vi "WILT Panel SS Station Labels.vi"(10 "Label Com Array":string[][](array[string])=[["M1", "100"], ["M3", "3"], ["M5", "5"], ["M7", "7"], ["M9", "9"], ["M11", "11"], ["M13", "13"], ["M15", "15"], ["M17", "17"], ["M19", "19"], ["M2", "2"], ["M4", "4"], ["M6", "6"], ["M8", "8"], ["M10", "10"], ["M12", "12"], ["M14", "14"], ["M16", "16"], ["M18", "18"], ["M20", "20"], ["N6", "21"], ["N7", "22"], ["N8", "23"], ["N9", "24"], ["N10", "25"], ["N11", "26"], ["N12", "27"], ["N13", "28"]]) -> (2 "Array Out":string[][](array[string]))   [LabVIEW 2016]
panel:
  in  "Complete":bool
  in  "Station A":string="DGnn"
  in  "Station C":string="58,50"
  in  "Station D":string="GE HEWH 1"
  in  "Station B":string="HEWH-MAN_OV"
  # "Enter Station Labels"
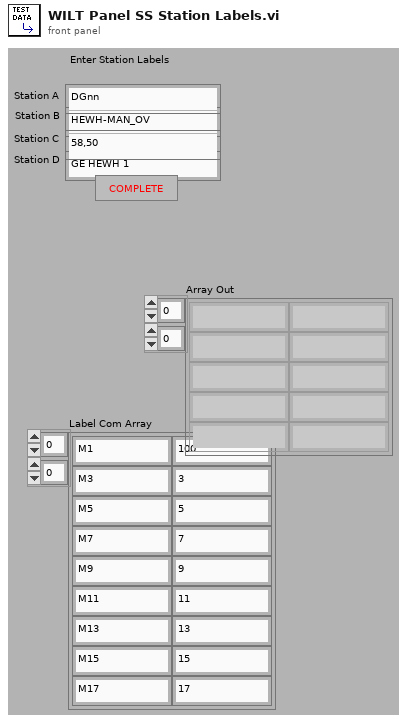
[diagram p1: front panel]
types:
  T1 = cluster{"Label Com Array[0]":string, "Label Com Array[1]":string, "Label Com Array[2]":string, "Label Com Array[3]":string}
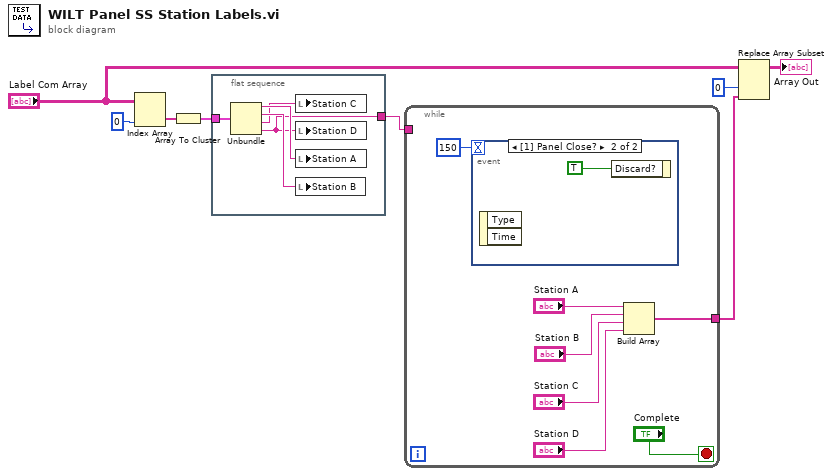
[diagram p0: block diagram]
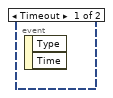
[diagram p2: hidden frame]
diagram:
  n1 = Index Array(array="Label Com Array", index (col)=0 ("disabled index (col)")) -> (element=w6:string[])  [unwired: 1 in]
  n2 = Array To Cluster(array=w6) -> (cluster=w8:T1)
  n3 = flat-sequence {
    tunnel: w8 -> [w13]
    tunnel: [w9] -> w5
    frame #0 {
      n4 = Unbundle(w13) -> ("Label Com Array[0]"=w12:string, "Label Com Array[1]"=w11:string, "Label Com Array[2]"=w10:string, "Label Com Array[3]"=w9:string)
      n5 = local write "Station C"(w10) -> ()
      n6 = local write "Station D"(w9) -> ()
      n7 = local write "Station A"(w12) -> ()
      n8 = local write "Station B"(w11) -> ()
    }
  }
  n9 = while {
    tunnel: w5 -> [_]
    tunnel: [w15] -> w3
    stop <- "Complete" stop-if-true
    n10 = event shown="[1] Panel Close?" {
      selector: _ -> [_ _]
      dyn-events: _ -> [_ _]
      timeout: u32 150 ("milliseconds to wait") -> [_ _]
      event Timeout {
        n11 = event-data() -> ()  [unwired: 1 in, 2 out]
      }
      event Panel Close? {
        n12 = event-data() -> ()  [unwired: 1 in, 2 out]
        n13 = event-data("Discard?"=TRUE) -> ()  [unwired: 1 in, 1 out]
      }
    }
    n14 = Build Array("Station A", "Station B", "Station C", "Station D") -> (w15:string[])
  }
  n15 = Replace Array Subset(array="Label Com Array", new element=w3, index (col)=0 ("disabled index (col)")) -> (→"Array Out":string[][])  [unwired: 1 in]
